vi "ZK注射泵系数读取.vi"(7 "是否启用通讯通知":bool, 8 "error in (no error)":errorcluster, 11 "Slave ID":T1) -> (0 "error out":errorcluster, 2 "B":sgl, 3 "K":sgl)   [LabVIEW 2016, in "质控单元V4.lvlib"]
uses:
  <vilib>/Plasmionique/MB Master/MB_Master/MB_Master.lvclass
  <vilib>/Plasmionique/MB Master/MB Master.lvlib
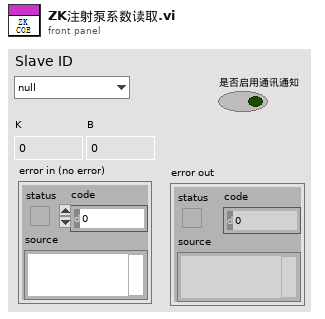
[diagram p1: front panel]
types:
  T1 = typedef "质控单元V4.lvlib/质控slave id.ctl" = enum16{"null", "氨氮", "总磷", "总氮", "CODMn", "CODCr", "氟化物", "挥发酚"}
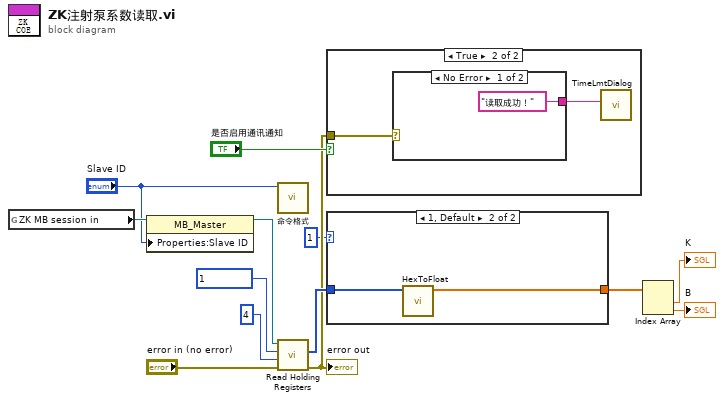
[diagram p0: block diagram]
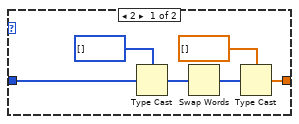
[diagram p2: hidden frame]
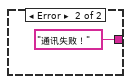
[diagram p4: hidden frame]
diagram:
  n1 = global read "ZK非断电保存全局变量.vi" "ZK MB session in"() -> (w12:refnum<class "MB_Master.lvclass">)
  n2 = property class="MB_Master"(reference=w12, "Properties:Slave ID"="Slave ID") -> (reference out=w10:refnum<class "MB_Master.lvclass">)  [unwired: 1 in, 1 out]
  n3 = call "命令格式.vi"("站号"="Slave ID") -> ()  [unwired: 10 in, 1 out]
  n4 = call <vilib>:"Read Holding Registers.vi"("error in (no error)"="error in (no error)", "quantity"=u16 4, "starting address"=u16 1, "MB session in"=w10) -> ("error out"=w3:errorcluster, "Registers"=w8:u16[])  [unwired: 5 in, 1 out]
  "error out" <- w3
  n5 = case shown="True" "是否启用通讯通知" {
    tunnel: w3 -> [_ w15]
    frame False {
    }
    frame True {
      n6 = case shown="No Error" w15 {
        tunnel: ["读取成功！" "通讯失败！"] -> w14
        frame No Error {
        }
        frame Error {
        }
      }
      n7 = call "TimeLmtDialog.vi"("Infoin"=w14) -> ()  [unwired: 11 in]
    }
  }
  n8 = case shown="1, Default" u16 1 ("命令格式") {
    tunnel: w8 -> [w22 w25]
    tunnel: [w18 w24] -> w7
    frame 2 {
      n9 = Type Cast(type=u32[] [], x=w22) -> (*(type *) &x=w21:u32[])
      n10 = Swap Words(1:w21) -> (0:w20:u32[])
      n11 = Type Cast(type=sgl[] [], x=w20) -> (*(type *) &x=w18:sgl[])
    }
    frame 1, Default {
      n12 = call "HexToFloat.vi"("数组"=w25) -> ("FLOAT"=w24:sgl[])  [unwired: 10 in]
    }
  }
  n13 = Index Array(array=w7) -> (element #1=→"K":sgl, element #2=→"B":sgl)  [unwired: 2 in]
